vi "LVClass_CorrectionDataManager GetExperienceCommands.vi"(0 "CorrectionDataManager in":refnum<class "CorrectionDataManager.lvclass">, 5 "N° actuator":i32, 11 "error in (no error)":errorcluster) -> (4 "CorrectionDataManager out":refnum<class "CorrectionDataManager.lvclass">, 8 "First DeltaCommand":sgl[](array[numeric]), 10 "Second DeltaCommand":sgl[](array[numeric]), 15 "error out":errorcluster)   [LabVIEW 2020, in "CorrectionDataManager.lvclass"]
doc: "Get the two wavefront corrector commands corresponding to the actuator\nactuator_index calibration.\n\n<B>corrdata_managerIn</B> : CorrDataManager object.\n<B>corrdata_managerOut</B> : CorrDataManager object.\n<B>actuator_index</B> : Index of the actuator.\n<B>first_command</B> : Wavefront corrector commands associated to the first move (push / positive\n displacement) of index actuator calibration.\n<B>second_command</B> : Wavefront corrector commands associated to the second move (pull / negative\n displacement) of index actuator calibration."
uses:
  CorrectionDataManager.lvclass
  CorrectionDataManager.lvclass/CorrectionDataManager.ctl
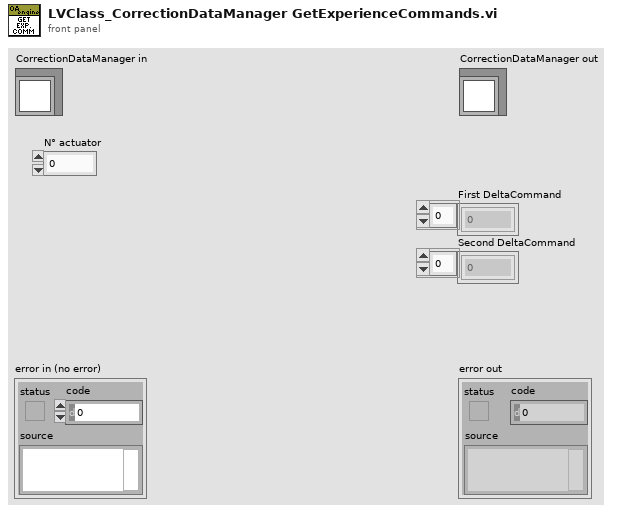
[diagram p1: front panel]
types:
  T1 = typedef "ClassID.ctl" = i64
  T2 = typedef "Wavefront Corrector states - ONE.ctl" = cluster{"Max":sgl, "Min":sgl, "Validity":enum16{"valid", "fixed", "invalid"}, "Fixed_Position":sgl}
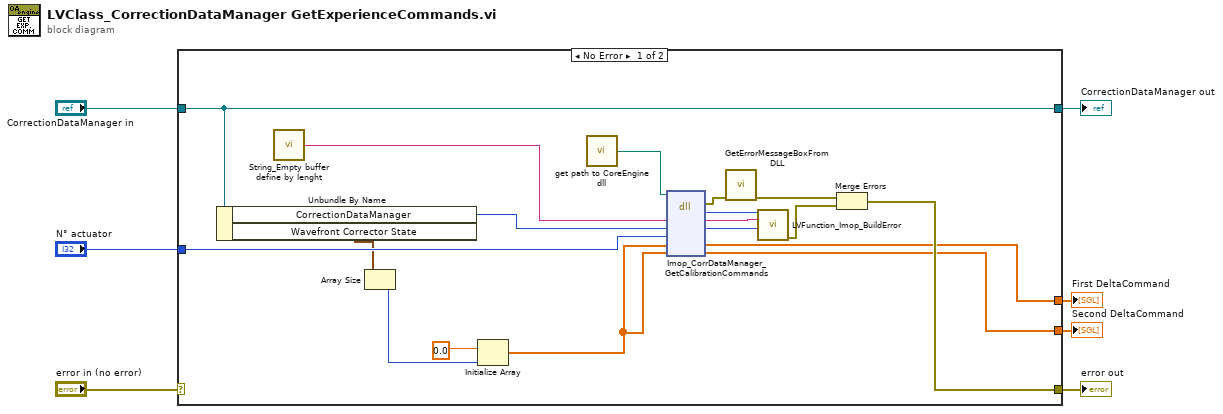
[diagram p0: block diagram]
diagram:
  n1 = case shown="No Error" "error in (no error)" {
    selector: "error in (no error)" -> [_ w27]
    tunnel: [w18 w27] -> w7
    tunnel: [w16 w26] -> w6
    tunnel: "CorrectionDataManager in" -> [w16 w26]
    tunnel: "N° actuator" -> [w15 _]
    tunnel: [w14 _] -> w2
    tunnel: [w13 _] -> w1
    frame No Error {
      n2 = Unbundle By Name(w16) -> ("CorrectionDataManager"=w17:T1, "Wavefront Corrector State"=w12:T2[])
      n3 = call "String_Empty buffer define by lenght.vi"() -> ("Empty buffer"=w23:string)  [unwired: 1 in]
      n4 = Array Size(array=w12) -> (size(s)=w11:i32)
      n5 = Initialize Array(sgl 0.0, w11) -> (w9:sgl[])
      n6 = call "get path to CoreEngine dll.vi"() -> ("path to wavekit library"=w22:path)  [unwired: 14 in, 1 out]
      n7 = dll-call lib="D:/soft/HASO_v3/SVN_trunk/ImOpCoreEngine4_LV2011/DLLs/c_interface_vc100.dll" fn="Imop_CorrDataManager_GetCalibrationCommands"(path in=w22, "message"=w23, "corrdata_manager"=w17, "experience_index"=w15, "First command_push_positive"=w9, "Second command_pull_negative"=w9) -> (error out=w21:errorcluster, "return type"=w25:i32, "message"=w24:string, "corrdata_manager"=w8:i64, "First command_push_positive"=w14:sgl[], "Second command_pull_negative"=w13:sgl[])  [unwired: 3 in, 1 out]
      n8 = call "GetErrorMessageBoxFromDLL.vi"("error IN"=w21) -> ("error OUT"=w20:errorcluster)  [unwired: 10 in]
      n9 = call "LVFunction_Imop_BuildError.vi"("code"=w25, "String to Prepend to source (\"\")"=w24, "Adresse"=w8) -> ("error out"=w19:errorcluster)  [unwired: 12 in]
      n10 = Merge Errors(w20, w19) -> (w18:errorcluster)
    }
    frame Error {
    }
  }
  "error out" <- w7
  "CorrectionDataManager out" <- w6
  "First DeltaCommand" <- w2
  "Second DeltaCommand" <- w1
